vi "Autonomous Independent.vi"() -> ()   [LabVIEW 2014]
doc: "This VI is called when autonomous begins, and will automatically be terminated when autonomous ends. You can carry out timed or sensor driven robot movement independently without needing to return to the caller."
uses:
  <vilib>/Rock Robotics/WPI/Joystick/WPI_JoystickGetSetRefNum.vi
  <vilib>/Rock Robotics/Network Tables/SD Write Numeric Array.vi
  <vilib>/Rock Robotics/WPI/RobotDrive/WPI_RobotDriveGetSetRefNum.vi
  Robot Global Data.vi
  <vilib>/Rock Robotics/WPI/RobotDrive/WPI_RobotDriveMecanumDrive_Cartesian.vi
panel:
  out "Current Movement, for debugging":T1 {"Z Joystick Value" scale=-1.0..1.0; "Y Joystick Value" scale=1.0..-1.0; "X Joystick Value" scale=-1.0..1.0}
  in  "Array of robot movements":T2(array[cluster]) {"Z Joystick Value" scale=-1.0..1.0; "Y Joystick Value" scale=1.0..-1.0; "X Joystick Value" scale=-1.0..1.0}
  # "Be sure to right-click and choose Data Operations>>Make Current Value default if you want to save the array values with the VI"
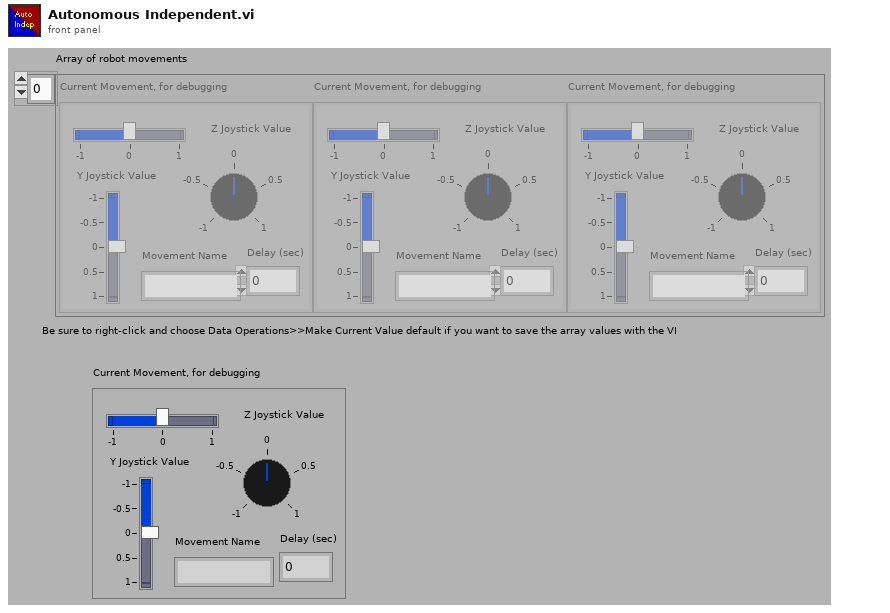
[diagram p1: front panel]
types:
  T1 = cluster{"X Joystick Value":dbl, "Y Joystick Value":dbl, "Z Joystick Value":dbl, "Delay (sec)":dbl, "Movement Name":string}
  T2 = cluster{"X Joystick Value":dbl, "Y Joystick Value":dbl, "Z Joystick Value":dbl, "Delay (sec)":dbl, "Movement Name":string}[]
  T3 = typedef "WPI_JoystickDevRef.ctl" = cluster{"Device":T4}
  T4 = typedef "WPI_JoystickDeviceEnum.ctl" = enum16{"USB 0", "USB 1", "USB 2", "USB 3", "USB 4", "USB 5"}
  T5 = typedef "WPI_RobotDriveDevRef.ctl" = cluster{"DevStatus":errorcluster, "Motors[]":T6[], "Square Inputs":bool, "Max Output":dbl}
  T6 = typedef "WPI_MotorControlDeviceRef.ctl" = cluster{"DeviceStatus":errorcluster, "Type":T7, "PWM":cluster{"Controller":T8, "PWM Channel":T9, "DeadBand":T10}, "CAN":cluster{"Device Number":u8, "Control Mode":T11, "Semaphore":T12, "Max Vout":dbl, "TalonSRX Control Mode":T13}, "Invert":bool, "TransformRef":T14, "InvTransformRef":T14}
  T7 = typedef "WPI_MotorControlType.ctl" = enum16{"PWM", "CAN", "CANTalonSRX"}
  T8 = typedef "FPGA_TypedefDigitalModule.ctl" = enum16{"Controller 1"}
  T9 = typedef "FPGA_DIOPWMChannel.ctl" = enum8{"PWM 0", "PWM 1", "PWM 2", "PWM 3", "PWM 4", "PWM 5", "PWM 6", "PWM 7", "PWM 8", "PWM 9", "PWM MXP 0", "PWM MXP 1", "PWM MXP 2", "PWM MXP 3", "PWM MXP 4", "PWM MXP 5", "PWM MXP 6", "PWM MXP 7", "PWM MXP 8", "PWM MXP 9", "Invalid"}
  T10 = typedef "WPI_PWMDeadband.ctl" = cluster{"Name":string, "maxPositivePwm":i32, "minPositivePwm":i32, "centerPwm":i32, "maxNegativePwm":i32, "minNegativePwm":i32, "angularRange":u16}
  T11 = typedef "WPI_CANJaguar_ControlMode.ctl" = enum8{"Percent VBus", "Current", "Speed", "Position", "Voltage"}
  T12 = typedef "Semaphore RefNum" = refnum<k1>
  T13 = typedef "WPI_CANTalonSRX_APIControlMode.ctl" = enum8{"Percent VBus", "Speed", "Position", "Slave", "Unchanged / Invalid"}
  T14 = typedef "WPI_PWMTransform_ConPane.ctl" = refnum<vi>
  T15 = typedef "WPI_EncoderDevRef.ctl" = cluster{"DevStatus":errorcluster, "EncoderIndex":T16, "CounterIndex":T17, "DistancePerCount":dbl, "Decoding Type":T18}
  T16 = typedef "FPGA_EncoderIdx.ctl" = enum8{"Enc 0", "Enc 1", "Enc 2", "Enc 3", "Enc 4", "Enc 5", "Enc 6", "Enc 7", "Invalid"}
  T17 = typedef "FPGA_CounterCtrSystemIndex.ctl" = enum8{"Ctr 0", "Ctr 1", "Ctr 2", "Ctr 3", "Ctr 4", "Ctr 5", "Ctr 6", "Ctr 7", "Invalid"}
  T18 = typedef "WPI_EncoderType.ctl" = enum16{"1x", "2x", "4x"}
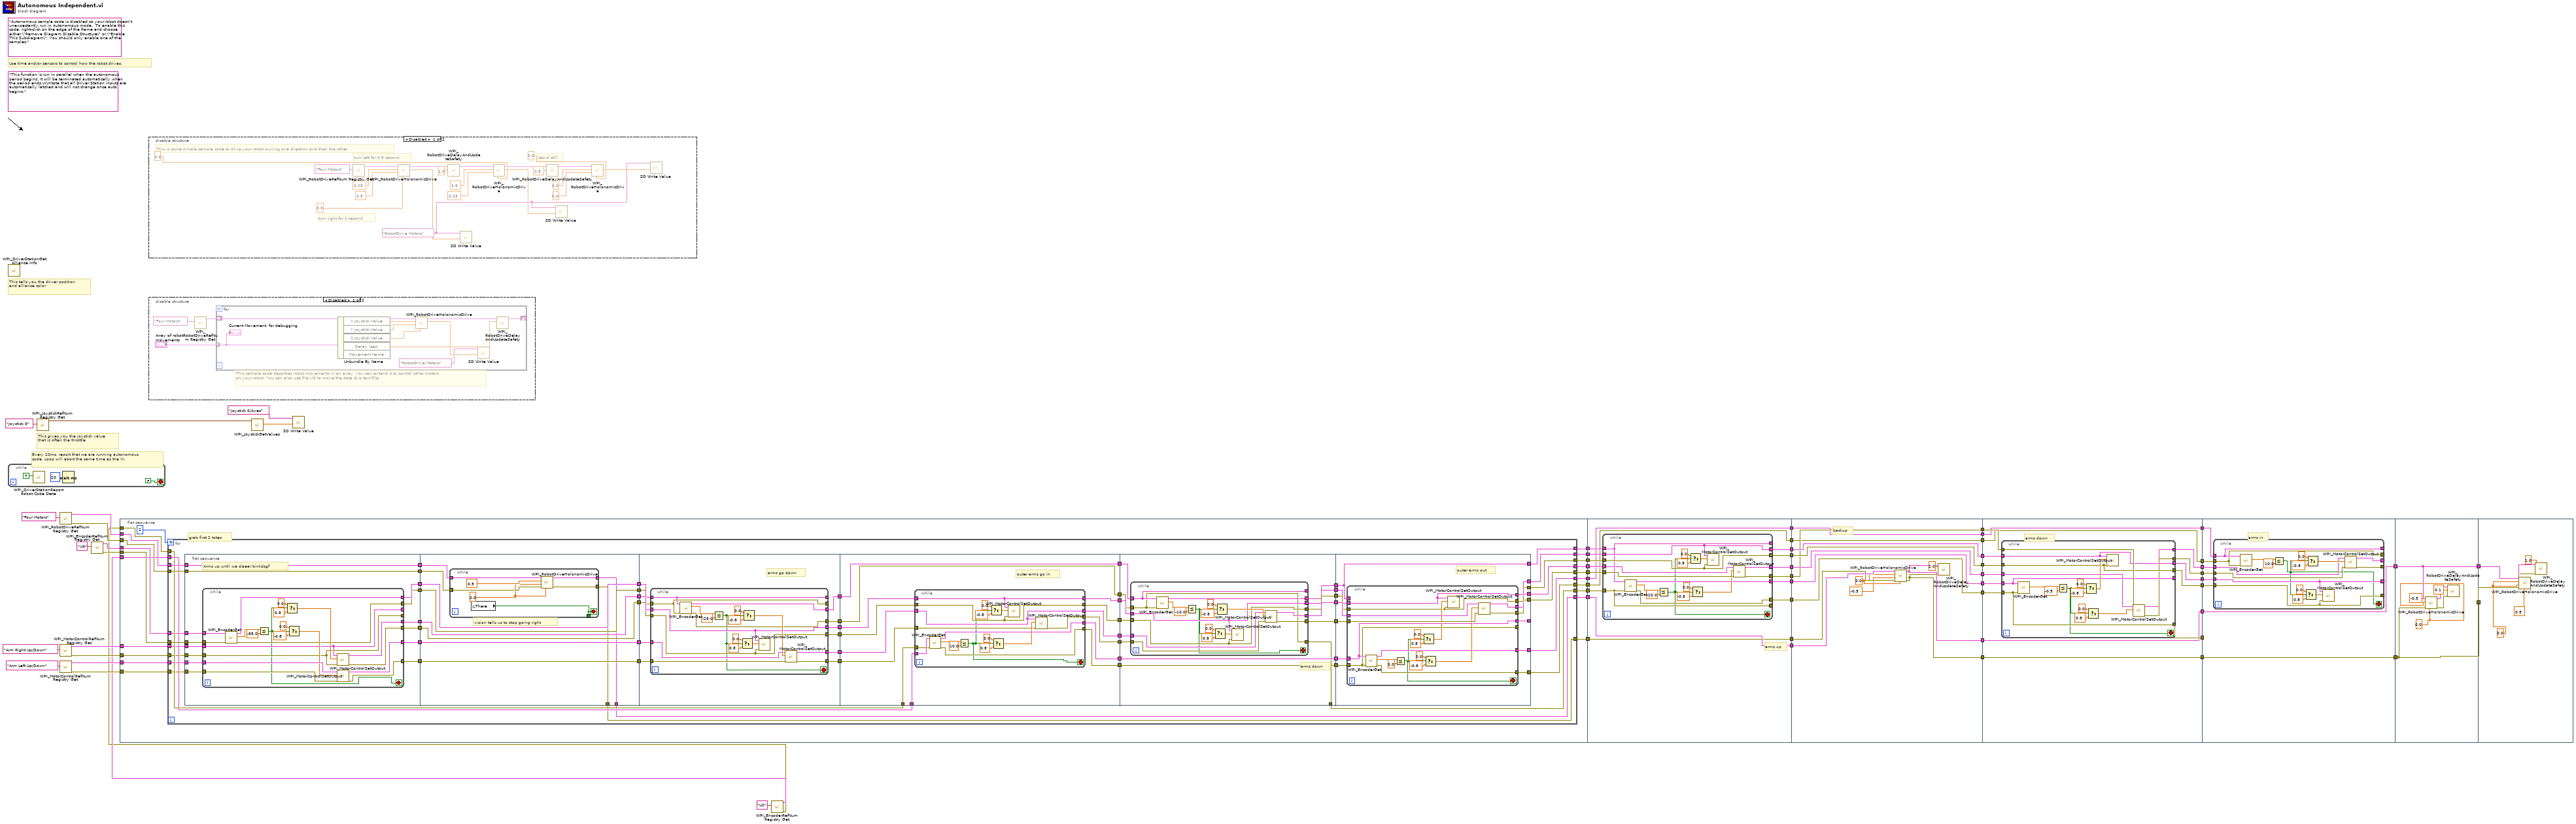
[diagram p0: block diagram]
diagram:
  (unwired) "Autonomous sample code is disabled so your robot doesn't unexpectantly run in Autonomous mode.  To enable this code, right-click on the edge of the frame and choose either \"Remove Diagram Disable Structure\" or \"Enable This Subdiagram\". You should only enable one of the samples."
  (unwired) "This function is run in parallel when the autonomous period begins. It will be terminated automatically when the period ends.\n\nNote that all Driver Station inputs are automatically latched and will not change once auto begins."
  # "Every 20ms, report that we are running autonomous\ncode. Loop will abort the same time as the VI."
  # "This gives you the joystick value\nthat is often the throttle"
  # "Use time and/or sensors to control how the robot drives."
  # "This tells you the driver position\nand alliance color"
  n1 = call <vilib>:"WPI_DriverStationGet Alliance Info.vi"() -> ()  [unwired: 12 out]
  n2 = while {
    stop <- FALSE stop-if-true
    n3 = call <vilib>:"WPI_DriverStationReport Robot Code State.vi"("Autonomous"=TRUE) -> ()  [unwired: 10 in, 1 out]
    n4 = Wait (ms)(milliseconds to wait=u32 20) -> ()  [unwired: 1 out]
  }
  n5 = call <vilib>:"WPI_JoystickRefNum Registry Get.vi"("refnum name"="Joystick 0") -> ("JoystickDevRef"=w61:T3)  [unwired: 1 in, 9 out]
  n6 = call <vilib>:"WPI_RobotDriveRefNum Registry Get.vi"("refnum name"="Four Motors") -> ("error out"=w52:errorcluster, "RobotDriveDevRef"=w53:T5)  [unwired: 1 in, 8 out]
  n7 = call <vilib>:"WPI_MotorControlRefNum Registry Get.vi"("refnum name"="Arm Right Up/Down") -> ("error out"=w50:errorcluster, "MotorControlDevRef"=w51:T6)  [unwired: 9 in]
  n8 = call <vilib>:"WPI_MotorControlRefNum Registry Get.vi"("refnum name"="Arm Left Up/Down") -> ("error out"=w46:errorcluster, "MotorControlDevRef"=w47:T6)  [unwired: 9 in]
  n9 = call <vilib>:"WPI_EncoderRefNum Registry Get.vi"("refnum name"="VR") -> ("error out"=w48:errorcluster, "EncoderDevRef"=w49:T15)  [unwired: 9 in]
  n10 = flat-sequence {
    tunnel: w53 -> [w86]
    tunnel: w52 -> [w85]
    tunnel: w51 -> [w84]
    tunnel: w50 -> [w83]
    tunnel: w49 -> [w82]
    tunnel: w48 -> [w81]
    tunnel: w47 -> [w80]
    tunnel: w46 -> [w79]
    tunnel: w45 -> [w78]
    tunnel: w44 -> [w77]
    tunnel: [w75] -> w43
    tunnel: [w74] -> w42
    tunnel: [w73] -> w41
    tunnel: [w72] -> w40
    tunnel: [w71] -> w39
    tunnel: [w70] -> w38
    tunnel: [w69] -> w37
    tunnel: [w68] -> w34
    tunnel: [w67] -> w18
    tunnel: [w66] -> w15
    tunnel: w43 -> [w337]
    tunnel: w42 -> [w336]
    tunnel: w41 -> [w335]
    tunnel: w40 -> [w334]
    tunnel: w39 -> [w333]
    tunnel: w38 -> [w332]
    tunnel: w37 -> [w331]
    tunnel: [w331] -> w36
    tunnel: [w330] -> w35
    tunnel: w34 -> [w330]
    tunnel: [w329] -> w33
    tunnel: [w328] -> w30
    tunnel: [w327] -> w29
    tunnel: [w326] -> w26
    tunnel: [w325] -> w24
    tunnel: [w324] -> w22
    tunnel: w18 -> [w323]
    tunnel: [w323] -> w17
    tunnel: [w322] -> w16
    tunnel: w15 -> [w322]
    tunnel: w36 -> [w371]
    tunnel: w35 -> [w370]
    tunnel: w33 -> [w369]
    tunnel: [w369] -> w32
    tunnel: [w368] -> w31
    tunnel: w30 -> [w368]
    tunnel: w29 -> [w367]
    tunnel: [w367] -> w28
    tunnel: [w366] -> w27
    tunnel: w26 -> [w366]
    tunnel: [w365] -> w25
    tunnel: w24 -> [w365]
    tunnel: [w364] -> w23
    tunnel: w22 -> [w364]
    tunnel: [w363] -> w20
    tunnel: w17 -> [w363]
    tunnel: w16 -> [w362]
    tunnel: [w362] -> w13
    tunnel: [w358] -> w8
    tunnel: [w357] -> w6
    tunnel: w32 -> [w386]
    tunnel: w31 -> [w385]
    tunnel: w28 -> [w384]
    tunnel: w27 -> [w383]
    tunnel: w25 -> [w382]
    tunnel: w23 -> [w381]
    tunnel: [w380] -> w21
    tunnel: w20 -> [w379]
    tunnel: [w379] -> w19
    tunnel: [w378] -> w14
    tunnel: w13 -> [w378]
    tunnel: [w377] -> w12
    tunnel: [w376] -> w11
    tunnel: [w375] -> w10
    tunnel: [w374] -> w9
    tunnel: w8 -> [w373]
    tunnel: [w373] -> w7
    tunnel: w6 -> [w372]
    tunnel: [w372] -> w5
    tunnel: w21 -> [_]
    tunnel: w19 -> [w411]
    tunnel: w14 -> [w410]
    tunnel: w12 -> [w409]
    tunnel: w11 -> [w408]
    tunnel: w10 -> [w407]
    tunnel: w9 -> [w406]
    tunnel: w7 -> [w405]
    tunnel: [w405] -> w4
    tunnel: w5 -> [w404]
    tunnel: [w404] -> w2
    tunnel: w4 -> [w435]
    tunnel: [w435] -> w3
    tunnel: w2 -> [w434]
    tunnel: [w434] -> w1
    tunnel: w3 -> [w440]
    tunnel: w1 -> [w439]
    frame #0 {
      # "grab first 2 totes"
      n11 = for {
        N: 2 -> [_]
        tunnel: w86 -> [w107]
        tunnel: w85 -> [w106]
        tunnel: w81 -> [w105]
        tunnel: w78 -> [w104]
        tunnel: w77 -> [w103]
        tunnel: w80 -> [w102]
        tunnel: w79 -> [w101]
        tunnel: w83 -> [w100]
        tunnel: w84 -> [w99]
        tunnel: w82 -> [w98]
        tunnel: [w97] -> w75
        tunnel: [w96] -> w74
        tunnel: [w94] -> w73
        tunnel: [w93] -> w72
        tunnel: [w92] -> w71
        tunnel: [w91] -> w70
        tunnel: [w90] -> w69
        tunnel: [w89] -> w68
        tunnel: [w88] -> w67
        tunnel: [w87] -> w66
        n12 = flat-sequence {
          tunnel: w106 -> [w154]
          tunnel: w107 -> [w155]
          tunnel: [w155] -> w141
          tunnel: [w154] -> w140
          tunnel: w105 -> [w153]
          tunnel: w102 -> [w152]
          tunnel: w101 -> [w151]
          tunnel: w99 -> [w142]
          tunnel: w100 -> [w150]
          tunnel: [w149] -> w139
          tunnel: [w148] -> w138
          tunnel: [w147] -> w137
          tunnel: [w146] -> w136
          tunnel: [w145] -> w135
          tunnel: [w144] -> w134
          tunnel: w98 -> [w143]
          tunnel: w141 -> [w186]
          tunnel: w140 -> [w185]
          tunnel: [w184] -> w133
          tunnel: w139 -> [w184]
          tunnel: [w183] -> w132
          tunnel: w138 -> [w183]
          tunnel: [w182] -> w131
          tunnel: w137 -> [w182]
          tunnel: [w181] -> w130
          tunnel: w136 -> [w181]
          tunnel: w135 -> [w180]
          tunnel: [w180] -> w129
          tunnel: [w179] -> w128
          tunnel: w134 -> [w179]
          tunnel: [w178] -> w90
          tunnel: [w177] -> w89
          tunnel: w133 -> [w205]
          tunnel: w132 -> [w204]
          tunnel: w131 -> [w203]
          tunnel: w130 -> [w202]
          tunnel: w129 -> [w201]
          tunnel: w128 -> [w200]
          tunnel: [w199] -> w127
          tunnel: [w198] -> w126
          tunnel: [w197] -> w125
          tunnel: [w196] -> w124
          tunnel: [w195] -> w123
          tunnel: [w194] -> w122
          tunnel: w104 -> [w238]
          tunnel: w103 -> [w237]
          tunnel: w127 -> [w236]
          tunnel: w126 -> [w235]
          tunnel: w125 -> [w234]
          tunnel: w124 -> [w233]
          tunnel: [w225] -> w121
          tunnel: [w232] -> w120
          tunnel: w123 -> [w231]
          tunnel: [w231] -> w119
          tunnel: [w230] -> w118
          tunnel: w122 -> [w230]
          tunnel: [w229] -> w117
          tunnel: [w228] -> w116
          tunnel: [w227] -> w115
          tunnel: [w226] -> w114
          tunnel: w121 -> [w270]
          tunnel: w120 -> [w269]
          tunnel: w119 -> [w268]
          tunnel: w118 -> [w267]
          tunnel: w117 -> [w266]
          tunnel: w116 -> [w265]
          tunnel: [w264] -> w113
          tunnel: w115 -> [w264]
          tunnel: w114 -> [w263]
          tunnel: [w263] -> w112
          tunnel: [w262] -> w111
          tunnel: [w261] -> w110
          tunnel: [w260] -> w109
          tunnel: [w259] -> w108
          tunnel: [w258] -> w95
          tunnel: [w257] -> w93
          tunnel: w113 -> [w302]
          tunnel: w112 -> [w301]
          tunnel: w111 -> [w300]
          tunnel: w110 -> [w299]
          tunnel: w109 -> [w298]
          tunnel: w108 -> [w297]
          tunnel: [w296] -> w97
          tunnel: [w295] -> w96
          tunnel: [w294] -> _
          tunnel: w95 -> [w293]
          tunnel: [w293] -> w94
          tunnel: [w292] -> w92
          tunnel: [w291] -> w91
          tunnel: [w290] -> w88
          tunnel: [w289] -> w87
          frame #0 {
            # "Arms up until we claear binkdsgf"
            n13 = while {
              tunnel: w152 -> [w176]
              tunnel: w151 -> [w175]
              tunnel: [w163] -> _
              tunnel: [w164] -> _
              tunnel: w153 -> [w174]
              tunnel: w143 -> [w165]
              tunnel: w142 -> [w163]
              tunnel: w150 -> [w164]
              tunnel: [w162] -> w149
              tunnel: [w161] -> w148
              tunnel: [w160] -> w147
              tunnel: [w159] -> w146
              tunnel: [w158] -> w145
              tunnel: [w157] -> w144
              stop <- w156 stop-if-true
              n14 = call <vilib>:"WPI_EncoderGet.vi"("error in (no error)"=w174, "EncoderDevRef"=w165) -> ("error out"=w157:errorcluster, "Distance"=w168:dbl, "EncoderDevRef"=w158:T15)  [unwired: 4 in, 3 out]
              n15 = Less Or Equal?(x=w168, y=-85.0) -> (x <= y?=w156:bool)
              n16 = Select(t=0.0, s=w156, f=0.8 ("Output")) -> (s? t:f=w166:dbl)
              n17 = Select(t=0.0, s=w156, f=-0.8 ("Output")) -> (s? t:f=w167:dbl)
              n18 = call <vilib>:"WPI_MotorControlSetOutput.vi"("error in (no error)"=w164, "Output"=w166, "MotorControlDevRef"=w163) -> ("error out"=w159:errorcluster, "MotorControlDevRef"=w160:T6)  [unwired: 6 in, 1 out]
              n19 = call <vilib>:"WPI_MotorControlSetOutput.vi"("error in (no error)"=w175, "Output"=w167, "MotorControlDevRef"=w176) -> ("error out"=w161:errorcluster, "MotorControlDevRef"=w162:T6)  [unwired: 6 in, 1 out]
            }
          }
          frame #1 {
            # "vision tells us to stop going right"
            n20 = while {
              tunnel: w186 -> [w193]
              tunnel: w185 -> [w192]
              tunnel: [w189] -> w178
              tunnel: [w188] -> w177
              tunnel: [w187] -> _
              stop <- w187 stop-if-true
              w190 = 0.0 ("Rotation")
              n21 = global read "Robot Global Data.vi" "There"() -> (w187:bool)
              n22 = call-poly <vilib>:"WPI_RobotDriveHolonomicDrive.vi"("Rotation"=w190, "error in (no error)"=w192, "Y"=w190, "X"=0.5, "RobotDriveDevRef"=w193) -> ("error out"=w188:errorcluster, "RobotDriveDevRef"=w189:T5)  [unwired: 4 in, 1 out]
            }
          }
          frame #2 {
            # "arms go down"
            n23 = while {
              tunnel: w204 -> [w224]
              tunnel: w203 -> [w214]
              tunnel: w202 -> [w215]
              tunnel: [w213] -> _
              tunnel: [w214] -> w199
              tunnel: [w215] -> w198
              tunnel: w201 -> [w213]
              tunnel: [w211] -> _
              tunnel: w205 -> [w212]
              tunnel: w200 -> [w211]
              tunnel: [w210] -> w197
              tunnel: [w209] -> w196
              tunnel: [w208] -> w195
              tunnel: [w207] -> w194
              stop <- w206 stop-if-true
              n24 = call <vilib>:"WPI_EncoderGet.vi"("error in (no error)"=w211, "EncoderDevRef"=w213) -> ("error out"=w207:errorcluster, "Distance"=w218:dbl, "EncoderDevRef"=w208:T15)  [unwired: 4 in, 3 out]
              n25 = Less Or Equal?(x=w218, y=-25.0) -> (x <= y?=w206:bool)
              n26 = Select(t=0.0, s=w206, f=0.8 ("Output")) -> (s? t:f=w216:dbl)
              n27 = Select(t=0.0, s=w206, f=-0.8 ("Output")) -> (s? t:f=w217:dbl)
              n28 = call <vilib>:"WPI_MotorControlSetOutput.vi"("error in (no error)"=w215, "Output"=w216, "MotorControlDevRef"=w214) -> ()  [unwired: 6 in, 3 out]
              n29 = call <vilib>:"WPI_MotorControlSetOutput.vi"("error in (no error)"=w224, "Output"=w217, "MotorControlDevRef"=w212) -> ("error out"=w210:errorcluster, "MotorControlDevRef"=w209:T6)  [unwired: 6 in, 1 out]
            }
          }
          frame #3 {
            # "outer arms go in"
            n30 = while {
              tunnel: [w248] -> w225
              tunnel: [w247] -> w232
              tunnel: [w243] -> w227
              tunnel: [w241] -> w226
              tunnel: [w245] -> w228
              tunnel: w238 -> [w244]
              tunnel: w237 -> [w242]
              tunnel: w236 -> [w248]
              tunnel: w235 -> [w247]
              tunnel: w234 -> [w246]
              tunnel: w233 -> [w245]
              tunnel: [w240] -> w229
              stop <- w239 stop-if-true
              n31 = call <vilib>:"WPI_EncoderGet.vi"("error in (no error)"=w242, "EncoderDevRef"=w244) -> ("error out"=w241:errorcluster, "Distance"=w251:dbl, "EncoderDevRef"=w243:T15)  [unwired: 4 in, 3 out]
              n32 = Less Or Equal?(x=w251, y=10.0) -> (x <= y?=w239:bool)
              n33 = Select(t=0.0, s=w239, f=-0.8 ("Output")) -> (s? t:f=w249:dbl)
              n34 = Select(t=0.0, s=w239, f=0.8 ("Output")) -> (s? t:f=w250:dbl)
              n35 = call <vilib>:"WPI_MotorControlSetOutput.vi"("error in (no error)"=w247, "Output"=w249, "MotorControlDevRef"=w248) -> ()  [unwired: 6 in, 3 out]
              n36 = call <vilib>:"WPI_MotorControlSetOutput.vi"("error in (no error)"=w246, "Output"=w250, "MotorControlDevRef"=w245) -> ("error out"=w240:errorcluster)  [unwired: 6 in, 2 out]
            }
          }
          frame #4 {
            # "arms down"
            n37 = while {
              tunnel: w266 -> [w288]
              tunnel: w270 -> [w278]
              tunnel: w269 -> [w279]
              tunnel: [w277] -> _
              tunnel: [w278] -> w259
              tunnel: [w279] -> w260
              tunnel: w268 -> [w277]
              tunnel: [w273] -> w257
              tunnel: w265 -> [w276]
              tunnel: [w275] -> w261
              tunnel: [w274] -> w262
              tunnel: w267 -> [w273]
              tunnel: [w272] -> w258
              stop <- w271 stop-if-true
              n38 = call <vilib>:"WPI_EncoderGet.vi"("error in (no error)"=w273, "EncoderDevRef"=w277) -> ("Distance"=w282:dbl, "EncoderDevRef"=w272:T15)  [unwired: 4 in, 4 out]
              n39 = Less Or Equal?(x=w282, y=-10.0) -> (x <= y?=w271:bool)
              n40 = Select(t=0.0, s=w271, f=0.8 ("Output")) -> (s? t:f=w280:dbl)
              n41 = Select(t=0.0, s=w271, f=-0.8 ("Output")) -> (s? t:f=w281:dbl)
              n42 = call <vilib>:"WPI_MotorControlSetOutput.vi"("error in (no error)"=w279, "Output"=w280, "MotorControlDevRef"=w278) -> ()  [unwired: 6 in, 3 out]
              n43 = call <vilib>:"WPI_MotorControlSetOutput.vi"("error in (no error)"=w288, "Output"=w281, "MotorControlDevRef"=w276) -> ("error out"=w275:errorcluster, "MotorControlDevRef"=w274:T6)  [unwired: 6 in, 1 out]
            }
          }
          frame #5 {
            # "outer arms out"
            n44 = while {
              tunnel: w299 -> [w321]
              tunnel: w297 -> [w303]
              tunnel: w298 -> [w312]
              tunnel: [w311] -> w294
              tunnel: [w303] -> w296
              tunnel: [w312] -> w295
              tunnel: w302 -> [w311]
              tunnel: [w307] -> _
              tunnel: w300 -> [w310]
              tunnel: [w309] -> w291
              tunnel: [w308] -> w292
              tunnel: w301 -> [w307]
              tunnel: w293 -> [_]
              tunnel: [w306] -> w290
              tunnel: [w305] -> w289
              stop <- w304 stop-if-true
              n45 = call <vilib>:"WPI_EncoderGet.vi"("error in (no error)"=w307, "EncoderDevRef"=w311) -> ("error out"=w306:errorcluster, "Distance"=w315:dbl, "EncoderDevRef"=w305:T15)  [unwired: 4 in, 3 out]
              n46 = Less Or Equal?(x=w315, y=0.0) -> (x <= y?=w304:bool)
              n47 = Select(t=0.0, s=w304, f=0.8 ("Output")) -> (s? t:f=w313:dbl)
              n48 = Select(t=0.0, s=w304, f=-0.8 ("Output")) -> (s? t:f=w314:dbl)
              n49 = call <vilib>:"WPI_MotorControlSetOutput.vi"("error in (no error)"=w312, "Output"=w313, "MotorControlDevRef"=w303) -> ()  [unwired: 6 in, 3 out]
              n50 = call <vilib>:"WPI_MotorControlSetOutput.vi"("error in (no error)"=w321, "Output"=w314, "MotorControlDevRef"=w310) -> ("error out"=w309:errorcluster, "MotorControlDevRef"=w308:T6)  [unwired: 6 in, 1 out]
            }
          }
        }
      }
    }
    frame #1 {
      # "arms up"
      n51 = while {
        tunnel: w332 -> [w356]
        tunnel: w337 -> [w346]
        tunnel: w336 -> [w347]
        tunnel: [w345] -> _
        tunnel: [w346] -> w329
        tunnel: [w347] -> w328
        tunnel: w335 -> [w345]
        tunnel: [w341] -> _
        tunnel: w333 -> [w344]
        tunnel: [w343] -> w324
        tunnel: [w342] -> w325
        tunnel: w334 -> [w341]
        tunnel: [w340] -> w327
        tunnel: [w339] -> w326
        stop <- w338 stop-if-true
        n52 = call <vilib>:"WPI_EncoderGet.vi"("error in (no error)"=w341, "EncoderDevRef"=w345) -> ("error out"=w339:errorcluster, "Distance"=w350:dbl, "EncoderDevRef"=w340:T15)  [unwired: 4 in, 3 out]
        n53 = Less Or Equal?(x=w350, y=-20.0) -> (x <= y?=w338:bool)
        n54 = Select(t=0.0, s=w338, f=0.8 ("Output")) -> (s? t:f=w348:dbl)
        n55 = Select(t=0.0, s=w338, f=-0.8 ("Output")) -> (s? t:f=w349:dbl)
        n56 = call <vilib>:"WPI_MotorControlSetOutput.vi"("error in (no error)"=w347, "Output"=w348, "MotorControlDevRef"=w346) -> ()  [unwired: 6 in, 3 out]
        n57 = call <vilib>:"WPI_MotorControlSetOutput.vi"("error in (no error)"=w356, "Output"=w349, "MotorControlDevRef"=w344) -> ("error out"=w343:errorcluster, "MotorControlDevRef"=w342:T6)  [unwired: 6 in, 1 out]
      }
    }
    frame #2 {
      w360 = 0.0 ("Rotation")
      # "backup"
      n58 = call-poly <vilib>:"WPI_RobotDriveHolonomicDrive.vi"("Rotation"=w360, "error in (no error)"=w370, "Y"=-0.5 ("X"), "X"=w360, "RobotDriveDevRef"=w371) -> ("error out"=w357:errorcluster, "RobotDriveDevRef"=w358:T5)  [unwired: 4 in, 1 out]
      n59 = call <vilib>:"WPI_RobotDriveDelayAndUpdateSafety.vi"("error in (no error)"=w357, "Delay (s)"=2.0, "RobotDriveDevRef"=w358) -> ()  [unwired: 7 in, 2 out]
    }
    frame #3 {
      # "arms down"
      n60 = while {
        tunnel: w381 -> [w403]
        tunnel: w386 -> [w393]
        tunnel: w385 -> [w394]
        tunnel: [w392] -> _
        tunnel: [w393] -> w377
        tunnel: [w394] -> w376
        tunnel: w384 -> [w392]
        tunnel: [w388] -> w380
        tunnel: w382 -> [w391]
        tunnel: [w390] -> w374
        tunnel: [w389] -> w375
        tunnel: w383 -> [w388]
        stop <- w387 stop-if-true
        n61 = call <vilib>:"WPI_EncoderGet.vi"("error in (no error)"=w388, "EncoderDevRef"=w392) -> ("Distance"=w397:dbl)  [unwired: 4 in, 5 out]
        n62 = Less Or Equal?(x=w397, y=-0.5) -> (x <= y?=w387:bool)
        n63 = Select(t=0.0, s=w387, f=-0.8 ("Output")) -> (s? t:f=w395:dbl)
        n64 = Select(t=0.0, s=w387, f=0.8 ("Output")) -> (s? t:f=w396:dbl)
        n65 = call <vilib>:"WPI_MotorControlSetOutput.vi"("error in (no error)"=w394, "Output"=w395, "MotorControlDevRef"=w393) -> ()  [unwired: 6 in, 3 out]
        n66 = call <vilib>:"WPI_MotorControlSetOutput.vi"("error in (no error)"=w403, "Output"=w396, "MotorControlDevRef"=w391) -> ("error out"=w390:errorcluster, "MotorControlDevRef"=w389:T6)  [unwired: 6 in, 1 out]
      }
    }
    frame #4 {
      # "arms in"
      n67 = while {
        tunnel: w406 -> [w428]
        tunnel: w409 -> [w418]
        tunnel: w408 -> [w419]
        tunnel: [w417] -> _
        tunnel: [w418] -> _
        tunnel: [w419] -> _
        tunnel: w410 -> [w417]
        tunnel: [w413] -> _
        tunnel: w407 -> [w416]
        tunnel: [w415] -> _
        tunnel: [w414] -> _
        tunnel: w411 -> [w413]
        stop <- w412 stop-if-true
        n68 = call <vilib>:"WPI_EncoderGet.vi"("error in (no error)"=w413, "EncoderDevRef"=w417) -> ("Distance"=w422:dbl)  [unwired: 4 in, 5 out]
        n69 = Less Or Equal?(x=w422, y=10.0) -> (x <= y?=w412:bool)
        n70 = Select(t=0.0, s=w412, f=0.8 ("Output")) -> (s? t:f=w420:dbl)
        n71 = Select(t=0.0, s=w412, f=-0.8 ("Output")) -> (s? t:f=w421:dbl)
        n72 = call <vilib>:"WPI_MotorControlSetOutput.vi"("error in (no error)"=w419, "Output"=w420, "MotorControlDevRef"=w418) -> ()  [unwired: 6 in, 3 out]
        n73 = call <vilib>:"WPI_MotorControlSetOutput.vi"("error in (no error)"=w428, "Output"=w421, "MotorControlDevRef"=w416) -> ("error out"=w415:errorcluster, "MotorControlDevRef"=w414:T6)  [unwired: 6 in, 1 out]
      }
    }
    frame #5 {
      w429 = 0.0 ("Rotation")
      n74 = call-poly <vilib>:"WPI_RobotDriveHolonomicDrive.vi"("Rotation"=w429, "error in (no error)"=w434, "Y"=-0.5, "X"=w429, "RobotDriveDevRef"=w435) -> ("error out"=w431:errorcluster, "RobotDriveDevRef"=w432:T5)  [unwired: 4 in, 1 out]
      n75 = call <vilib>:"WPI_RobotDriveDelayAndUpdateSafety.vi"("error in (no error)"=w431, "Delay (s)"=0.1, "RobotDriveDevRef"=w432) -> ()  [unwired: 7 in, 2 out]
    }
    frame #6 {
      w436 = 0.0 ("Rotation")
      n76 = call-poly <vilib>:"WPI_RobotDriveHolonomicDrive.vi"("Rotation"=0.5, "error in (no error)"=w439, "Y"=w436, "X"=w436, "RobotDriveDevRef"=w440) -> ("error out"=w441:errorcluster, "RobotDriveDevRef"=w442:T5)  [unwired: 4 in, 1 out]
      n77 = call <vilib>:"WPI_RobotDriveDelayAndUpdateSafety.vi"("error in (no error)"=w441, "Delay (s)"=1.0, "RobotDriveDevRef"=w442) -> ()  [unwired: 7 in, 2 out]
    }
  }
  n78 = disable-structure shown="Disabled" {
    frame Disabled {
      w449 = "RobotDrive Motors" ("Name")
      # "This is some simple sample code to drive your robot curving one direction and then the other."
      # "stand still"
      # "turn left for 0.5 second"
      # "turn right for 1 second"
      n79 = call <vilib>:"WPI_RobotDriveRefNum Registry Get.vi"("refnum name"="Four Motors") -> ("RobotDriveDevRef"=w450:T5)  [unwired: 1 in, 9 out]
      n80 = call-poly <vilib>:"WPI_RobotDriveHolonomicDrive.vi"("Rotation"=0.0, "Y"=0.5 ("X axis value"), "X"=0.25 ("X axis value"), "RobotDriveDevRef"=w450) -> ("Motor Values"=w445:dbl[], "RobotDriveDevRef"=w457:T5)  [unwired: 5 in, 1 out]
      n81 = call <vilib>:"WPI_RobotDriveDelayAndUpdateSafety.vi"("Delay (s)"=1.0, "RobotDriveDevRef"=w457) -> ("RobotDriveDevRef 2"=w456:T5)  [unwired: 8 in, 1 out]
      n82 = call-poly <vilib>:"SD Write Value.vi"("Numeric Array"=w445, "Name"=w449) -> ()  [unwired: 8 in, 2 out]
      n83 = call-poly <vilib>:"WPI_RobotDriveHolonomicDrive.vi"("Rotation"=0.0, "Y"=0.25 ("X axis value"), "X"=0.5 ("X axis value"), "RobotDriveDevRef"=w456) -> ("Motor Values"=w444:dbl[], "RobotDriveDevRef"=w455:T5)  [unwired: 5 in, 1 out]
      n84 = call <vilib>:"WPI_RobotDriveDelayAndUpdateSafety.vi"("Delay (s)"=0.5, "RobotDriveDevRef"=w455) -> ("RobotDriveDevRef 2"=w454:T5)  [unwired: 8 in, 1 out]
      n85 = call-poly <vilib>:"SD Write Value.vi"("Numeric Array"=w444, "Name"=w449) -> ()  [unwired: 8 in, 2 out]
      n86 = call-poly <vilib>:"WPI_RobotDriveHolonomicDrive.vi"("Rotation"=0.0 ("X axis value"), "Y"=0.0 ("X axis value"), "X"=0.0 ("X axis value"), "RobotDriveDevRef"=w454) -> ("Motor Values"=w443:dbl[])  [unwired: 5 in, 2 out]
      n87 = call-poly <vilib>:"SD Write Value.vi"("Numeric Array"=w443, "Name"=w449) -> ()  [unwired: 8 in, 2 out]
    }
    frame Enabled {
    }
  }
  n88 = disable-structure shown="Disabled" {
    frame Disabled {
      # "This sample code describes robot movements in an array. You can extend it to control other motors\non your robot. You can also use file I/O to move the data to a text file."
      n89 = call <vilib>:"WPI_RobotDriveRefNum Registry Get.vi"("refnum name"="Four Motors") -> ("RobotDriveDevRef"=w465:T5)  [unwired: 1 in, 9 out]
      n90 = for {
        shift-right: [w473] -> _
        shift-left: w465 -> [w474]
        tunnel: "Array of robot movements" -> [w469] mode=indexing
        n91 = Unbundle By Name(w469) -> ("X Joystick Value"=w472:dbl, "Y Joystick Value"=w471:dbl, "Z Joystick Value"=w468:dbl, "Delay (sec)"=w470:dbl)  [unwired: 1 out]
        n92 = call-poly <vilib>:"WPI_RobotDriveHolonomicDrive.vi"("Rotation"=w468, "Y"=w471, "X"=w472, "RobotDriveDevRef"=w474) -> ("Motor Values"=w467:dbl[], "RobotDriveDevRef"=w475:T5)  [unwired: 5 in, 1 out]
        n93 = call-poly <vilib>:"SD Write Value.vi"("Numeric Array"=w467, "Name"="RobotDrive Motors") -> ()  [unwired: 8 in, 2 out]
        n94 = call <vilib>:"WPI_RobotDriveDelayAndUpdateSafety.vi"("Delay (s)"=w470, "RobotDriveDevRef"=w475) -> ("RobotDriveDevRef 2"=w473:T5)  [unwired: 8 in, 1 out]
        "Current Movement, for debugging" <- w469
      }
    }
    frame Enabled {
    }
  }
  n95 = call <vilib>:"WPI_JoystickGetValues.vi"("JoystickDevRef"=w61) -> ("Axes"=w59:dbl[])  [unwired: 6 in, 4 out]
  n96 = call-poly <vilib>:"SD Write Value.vi"("Numeric Array"=w59, "Name"="Joystick 0/Axes") -> ()  [unwired: 8 in, 2 out]
  n97 = call <vilib>:"WPI_EncoderRefNum Registry Get.vi"("refnum name"="LO") -> ("error out"=w44:errorcluster, "EncoderDevRef"=w45:T15)  [unwired: 9 in]
